vi "Test_050620.vi"() -> ()   [LabVIEW 2020]
panel:
  out "XY Graph":cluster{"time":dbl[], "amplitude":dbl[]}(graph)
  in  "length of signal":dbl
  in  "Graph display":u16(ring)=6 items=["1", "2", "3", "1*2", "1*3", "2*3", "1*2*3"]
  in  "frequency 3":dbl=1.0 format="%0.2p"
  in  "offset (deg) 3":dbl=90.0 format="%0.2p"
  in  "amplitude 3":dbl=1.0 format="%0.2p"
  in  "frequency 2":dbl=1.0 format="%0.2p"
  in  "offset (deg) 2":dbl format="%0.2p"
  in  "amplitude 2":dbl=1.0 format="%0.2p"
  in  "frequency":dbl=1.0 format="%0.2p"
  in  "offset (deg)":dbl format="%0.2p"
  in  "amplitude":dbl=1.0 format="%0.2p"
  in  "stop":bool
  in  "sampling":i32=1000
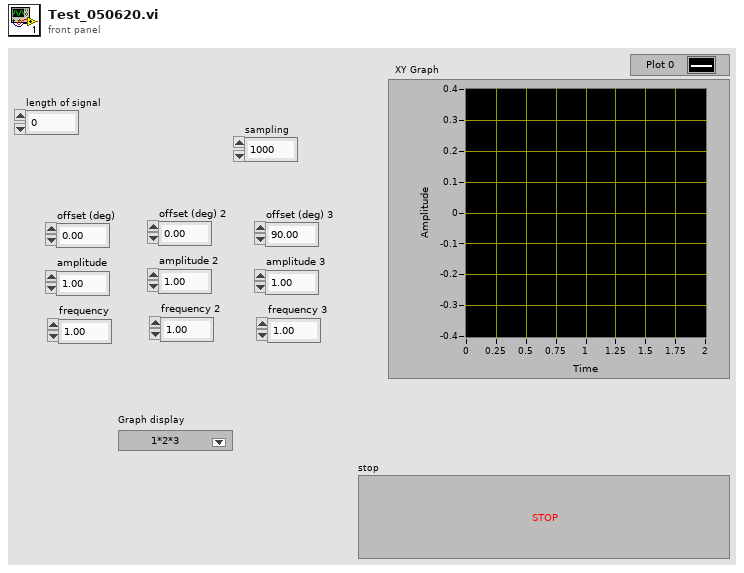
[diagram p1: front panel]
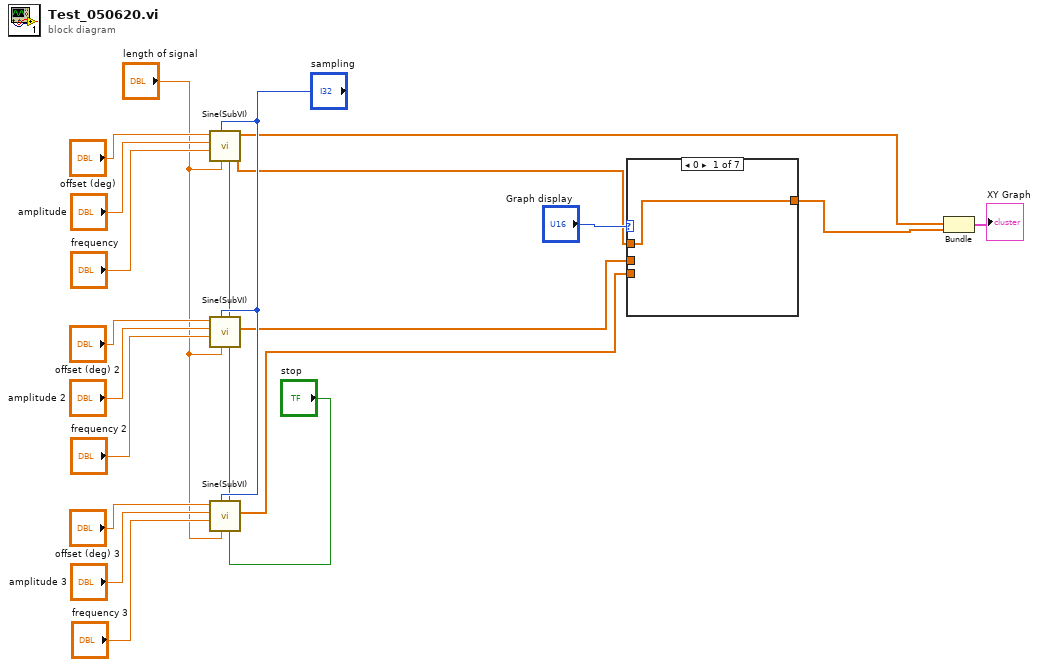
[diagram p0: block diagram]
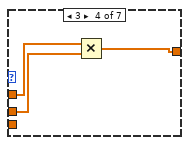
[diagram p4: hidden frame]
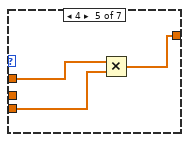
[diagram p5: hidden frame]
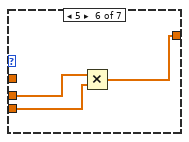
[diagram p6: hidden frame]
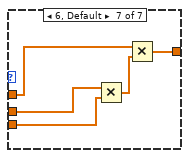
[diagram p7: hidden frame]
diagram:
  n1 = call "Sine(SubVI).vi"("stop"="stop", "length of signal"="length of signal", "sampling"="sampling", "frequency"="frequency", "amplitude"="amplitude", "offset (deg)"="offset (deg)") -> ("amplitude"=w6:dbl[], "time"=w2:dbl[])  [unwired: 4 in]
  n2 = call "Sine(SubVI).vi"("stop"="stop", "length of signal"="length of signal", "sampling"="sampling", "frequency"="frequency 2", "amplitude"="amplitude 2", "offset (deg)"="offset (deg) 2") -> ("amplitude"=w5:dbl[])  [unwired: 4 in, 1 out]
  n3 = call "Sine(SubVI).vi"("stop"="stop", "length of signal"="length of signal", "sampling"="sampling", "frequency"="frequency 3", "amplitude"="amplitude 3", "offset (deg)"="offset (deg) 3") -> ("amplitude"=w10:dbl[])  [unwired: 4 in, 1 out]
  n4 = case shown="0" "Graph display" {
    tunnel: w6 -> [w20 _ _ w25 w28 _ w34]
    tunnel: w5 -> [_ w21 _ w24 _ w31 w35]
    tunnel: w10 -> [_ _ w22 _ w27 w30 w36]
    tunnel: [w20 w21 w22 w23 w26 w29 w32] -> w3
    frame 0 {
    }
    frame 1 {
    }
    frame 2 {
    }
    frame 3 {
      n5 = Multiply(x=w25, y=w24) -> (x*y=w23:dbl[])
    }
    frame 4 {
      n6 = Multiply(x=w28, y=w27) -> (x*y=w26:dbl[])
    }
    frame 5 {
      n7 = Multiply(x=w31, y=w30) -> (x*y=w29:dbl[])
    }
    frame 6, Default {
      n8 = Multiply(x=w35, y=w36) -> (x*y=w33:dbl[])
      n9 = Multiply(x=w34, y=w33) -> (x*y=w32:dbl[])
    }
  }
  n10 = Bundle("time"=w2, "amplitude"=w3) -> (→"XY Graph":cluster{"time":dbl[], "amplitude":dbl[]})  [unwired: 1 in]
